vi "Fire_TTL_at_start_stop.vi"(8 "Serial Port":refnum<visa-resource-name>, 11 "Start/stop in":bool) -> (0 "Time to process command, ms":dbl, 3 "Start/stop out":bool)   [LabVIEW 2016]
doc: "Fires TTL High to the TTL2 output for ~250 ms."
uses:
  Globaltracker.vi
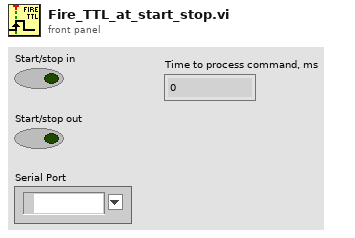
[diagram p1: front panel]
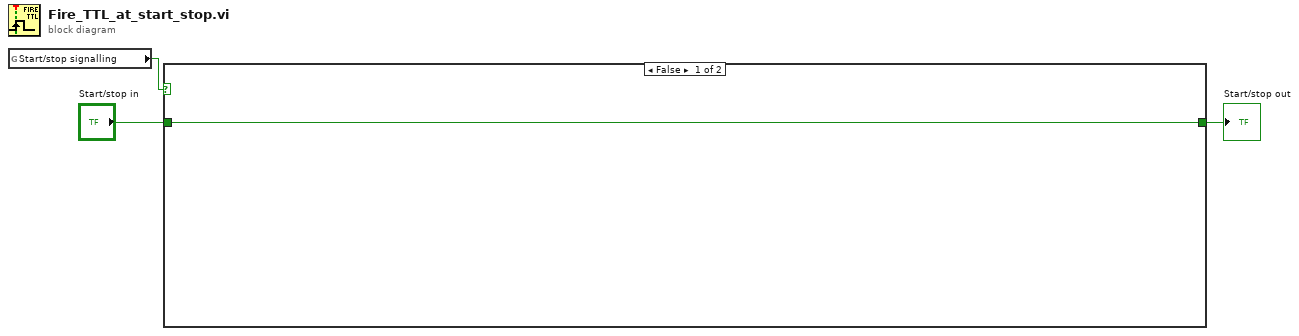
[diagram p0: block diagram]
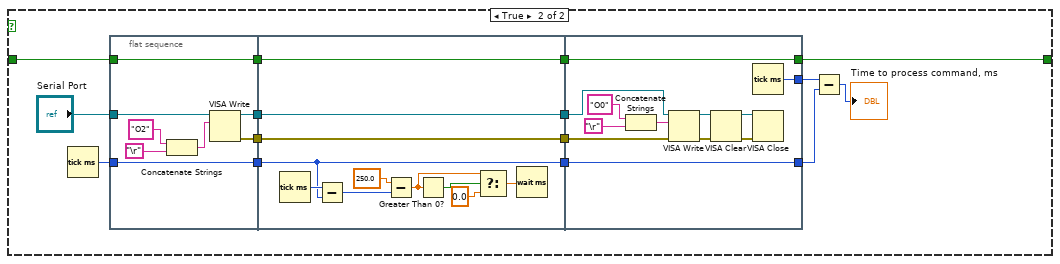
[diagram p2: hidden frame]
diagram:
  n1 = global read "Globaltracker.vi" "Start/stop signalling"() -> (w3:bool)
  n2 = case shown="False" w3 {
    tunnel: [w4 w6] -> w2
    tunnel: "Start/stop in" -> [w4 w5]
    frame False {
    }
    frame True {
      n3 = Tick Count (ms)() -> (millisecond timer value=w11:u32)
      n4 = flat-sequence {
        tunnel: "Serial Port" -> [w21]
        tunnel: [w24] -> w19
        tunnel: [w23] -> w18
        tunnel: [w22] -> w17
        tunnel: w5 -> [w22]
        tunnel: [w20] -> w12
        tunnel: w11 -> [w20]
        tunnel: [w38] -> w16
        tunnel: w19 -> [w38]
        tunnel: [w37] -> w15
        tunnel: w18 -> [w37]
        tunnel: w17 -> [w36]
        tunnel: [w36] -> w14
        tunnel: w12 -> [w28]
        tunnel: [w28] -> w8
        tunnel: w16 -> [w43]
        tunnel: w15 -> [w42]
        tunnel: w14 -> [w41]
        tunnel: [w41] -> w6
        tunnel: [w40] -> w10
        tunnel: [w39] -> w9
        tunnel: w8 -> [w39]
        frame #0 {
          n5 = Concatenate Strings("O2" ("string"), "\r") -> (w27:string)
          n6 = VISA Write(VISA resource name=w21, write buffer=w27) -> (VISA resource name out=w24:refnum<visa-resource-name>, error out=w23:errorcluster)  [unwired: 1 in, 1 out]
        }
        frame #1 {
          n7 = Tick Count (ms)() -> (millisecond timer value=w35:u32)
          n8 = Subtract(x=w35, y=w28) -> (x-y=w33:u32)
          n9 = Subtract(x=250.0, y=w33) -> (x-y=w30:dbl)
          n10 = Greater Than 0?(x=w30) -> (x > 0?=w32:bool)
          n11 = Select(t=w30, s=w32, f=0.0) -> (s? t:f=w31:dbl)
          n12 = Wait (ms)(milliseconds to wait=w31) -> ()  [unwired: 1 out]
        }
        frame #2 {
          n13 = Concatenate Strings("O0" ("string"), "\r") -> (w47:string)
          n14 = VISA Write(VISA resource name=w43, write buffer=w47, error in (no error)=w42) -> (VISA resource name out=w46:refnum<visa-resource-name>, error out=w45:errorcluster)  [unwired: 1 out]
          n15 = VISA Clear(VISA resource name=w46, error in (no error)=w45) -> (VISA resource name out=w50:refnum<visa-resource-name>, error out=w44:errorcluster)
          n16 = Tick Count (ms)() -> (millisecond timer value=w40:u32)
          n17 = VISA Close(VISA resource name=w50, error in (no error)=w44) -> ()  [unwired: 1 out]
        }
      }
      n18 = Subtract(x=w10, y=w9) -> (x-y=→"Time to process command, ms":u32)
    }
  }
  "Start/stop out" <- w2
